vi "DSF.Engine.Builder.Initialize VS Channels Array.vi"(8 "error in (no error)":errorcluster, 11 "Builder in":refnum<class "DSF.Engine.Builder.lvclass">) -> (0 "error out":errorcluster, 2 "VS Channels Array":dbl[](array[numeric]), 3 "Builder out":refnum<class "DSF.Engine.Builder.lvclass">)   [LabVIEW 2017, in "DSF.Engine.lvlib" / "DSF.Engine.Builder.lvclass"]
uses:
  DSF.Engine.Builder.lvclass
  Cache/DSF.Engine.Memory.Cache.Framework.lvclass
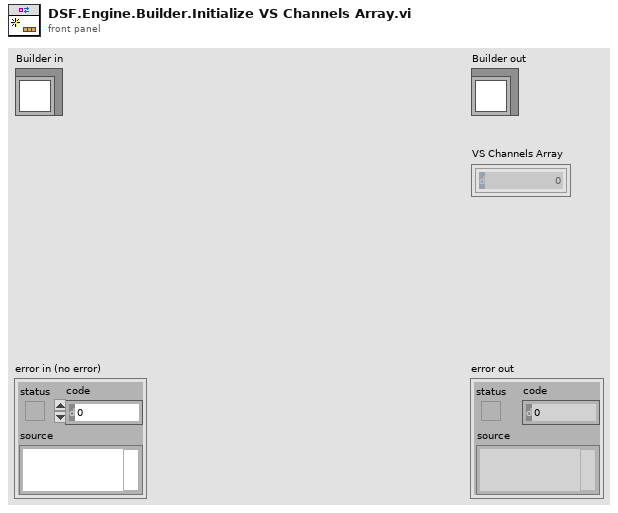
[diagram p1: front panel]
types:
  T1 = typedef "DSF.Shared.lvlib/DSF.Shared.Typedefs.Data Type Counts.ctl" = cluster{"Bool":u64, "SGL":u64, "DBL":u64, "I8":u64, "I16":u64, "I32":u64, "I64":u64, "U8":u64, "U16":u64, "U32":u64, "U64":u64}
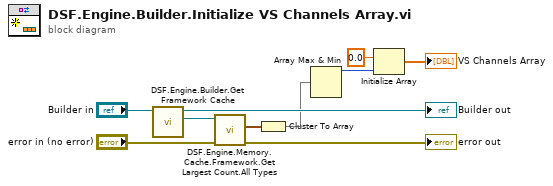
[diagram p0: block diagram]
diagram:
  n1 = call "DSF.Engine.Builder.Get Framework Cache.vi"("Builder in"="Builder in") -> ("Framework Cache"=w9:refnum<class "DSF.Engine.Memory.Cache.Framework.lvclass">, "Builder out"=→"Builder out":refnum<class "DSF.Engine.Builder.lvclass">)  [unwired: 9 in]
  n2 = call "DSF.Engine.Memory.Cache.Framework.Get Largest Count.All Types.vi"("error in (no error)"="error in (no error)", "Framework Cache in"=w9) -> ("error out"=→"error out":errorcluster, "Data Type Counts out"=w5:T1)  [unwired: 7 in, 1 out]
  n3 = Cluster To Array(cluster=w5) -> (array=w4:u64[])
  n4 = Array Max & Min(array=w4) -> (max value=w3:u64)  [unwired: 3 out]
  n5 = Initialize Array(0.0 ("element"), w3) -> (→"VS Channels Array":dbl[])
